vi "wrap.Call.vi"(0 "class.GLue in":refnum<class "class.GLue.lvclass">, 7 "NumArgs":i32, 11 "error in (no error)":errorcluster) -> (4 "class.GLue out":refnum<class "class.GLue.lvclass">, 8 "Return":i32, 13 "ErrString":string, 15 "error out":errorcluster)   [LabVIEW 2014, in "GLue.lvlib" / "class.GLue.lvclass"]
uses:
  class.GLue.lvclass
  class.GLue.lvclass/class.GLue.ctl
  Resources/GLue.dll
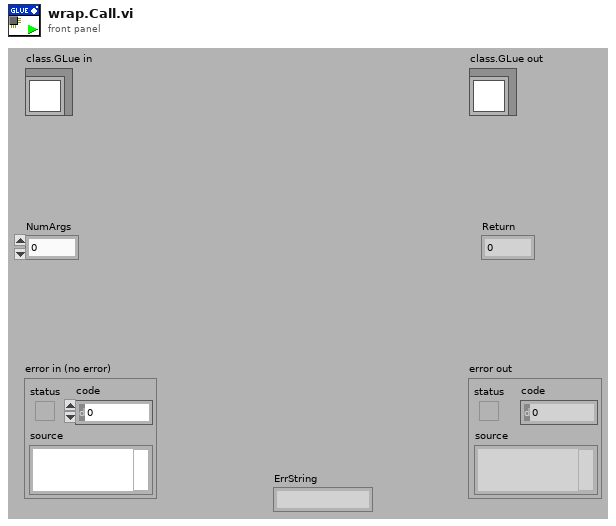
[diagram p1: front panel]
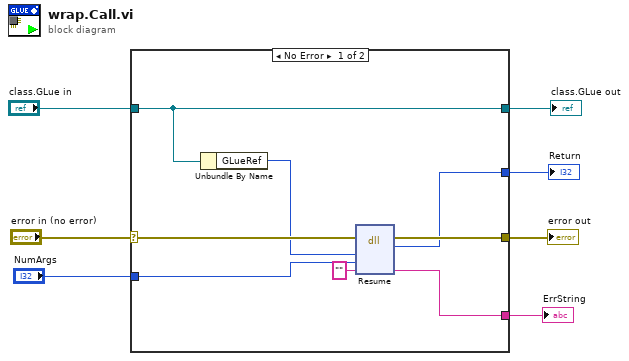
[diagram p0: block diagram]
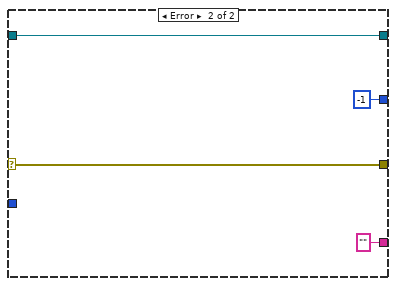
[diagram p2: hidden frame]
diagram:
  n1 = case shown="No Error" "error in (no error)" {
    selector: "error in (no error)" -> [w14 w19]
    tunnel: [w13 w19] -> w6
    tunnel: [w15 w18] -> w4
    tunnel: "class.GLue in" -> [w15 w18]
    tunnel: "NumArgs" -> [w11 _]
    tunnel: [w10 "" ("Error")] -> w2
    tunnel: [w8 -1 ("Return")] -> w1
    frame No Error {
      n2 = Unbundle By Name(w15) -> ("GLueRef"=w12:i64)
      n3 = dll-call lib="C:/Users/Antonie/Documents/work/glue/trunk/Resources/GLue.dll" fn="Resume"(error in=w14, "GLue"=w12, "NumArgs"=w11, "Error"="") -> (error out=w13:errorcluster, "Return"=w8:i32, "Error"=w10:string)  [unwired: 4 in, 1 out]
    }
    frame Error {
    }
  }
  "error out" <- w6
  "class.GLue out" <- w4
  "ErrString" <- w2
  "Return" <- w1
